vi "U3 AIN and PWM (ePut).vi"(9 "Timer0 Duty Cycle [%]":dbl=50.0 format="%.1f", 10 "16-bit PWM Frequency [Hz]":dbl=52.0 format="%.2f") -> (2 "Actual 16-bit Frequency":dbl format="%.1f")   [LabVIEW 2021]
panel:
  out "Timer0 Value":u16
  out "AIN0":dbl format="%_6g"
  in  "Timer/Counter Pin Offset":u8=4
  in  "stop":bool
  in  "FirstFound":bool=TRUE
  in  "Address":string="1"
  out "TimerClockDivisor":u8
  out "Error Message":string
  # "Demonstrates 1 channel of analog input with 1 channel of 16-bit PWM output.\nUses the 48 MHz divisor capable clock, and chooses a timer clock divisor to get\nas close as possible to the desired 16-bit PWM frequency.  Unlike \"U3 2-PWM.vi\",\nthis example updates the Timer0 Value every iteration even if it is the same.\nIf pin offset is 4, the PWM16 will be on FIO4."
  # "This example allows the duty cycle to\nbe changed while the VI is running."
  # "Range is 2.86 to 732.42 Hz"
  # "This VI passes a timer\nbase clock constant that\nis valid for hardware V1.21.\nFor hardware V1.20 change\nLJ_tc48MHZ_DIV to LJ_tc24MHZ_DIV."
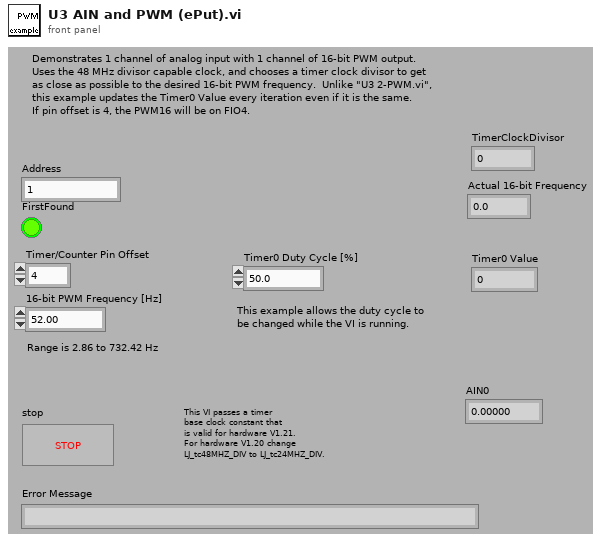
[diagram p1: front panel]
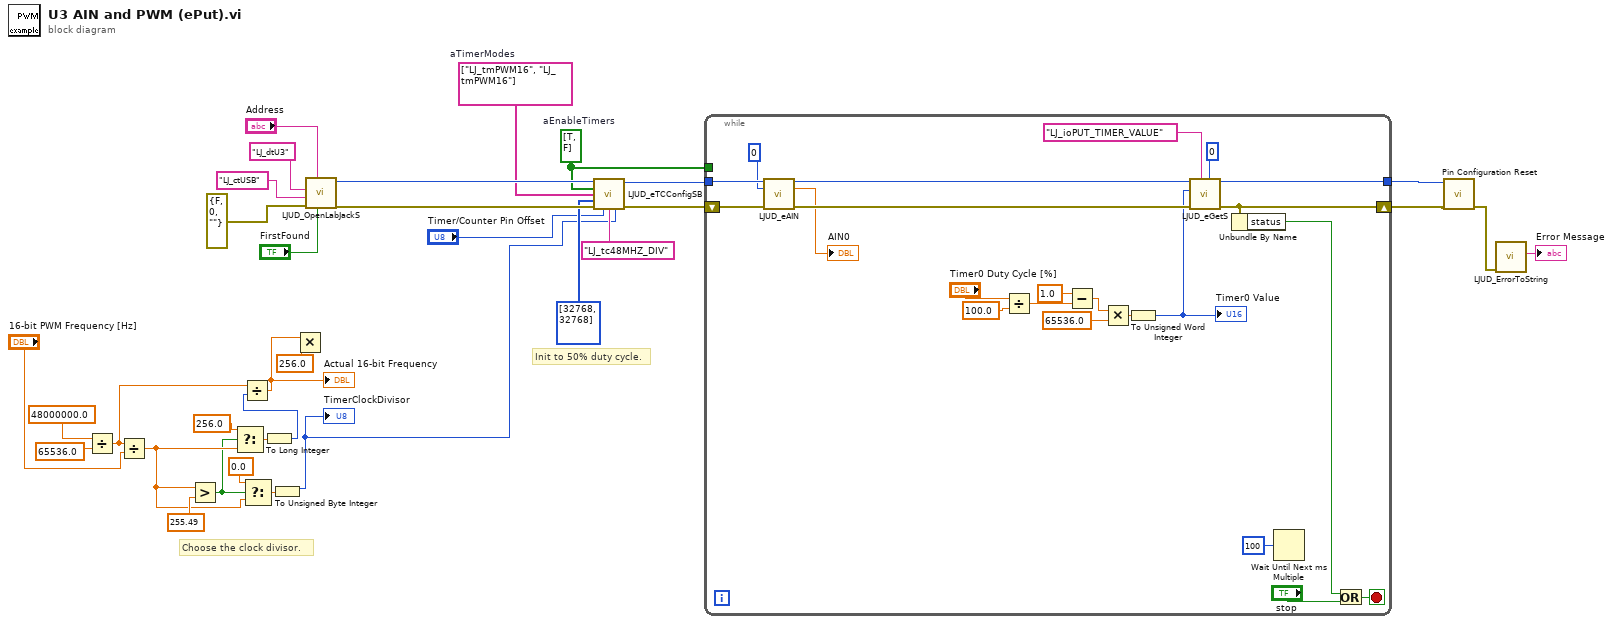
[diagram p0: block diagram]
diagram:
  w2 = bool[] [TRUE, FALSE]  # aEnableTimers
  w7 = string[] ["LJ_tmPWM16", "LJ_tmPWM16"]  # aTimerModes
  # "Choose the clock divisor."
  # "Init to 50% duty cycle."
  n1 = Divide(x=48000000.0, y=65536.0) -> (x/y=w21:dbl)
  n2 = Divide(x=w21, y="16-bit PWM Frequency [Hz]") -> (x/y=w25:dbl)
  n3 = Greater?(x=w25, y=255.49) -> (0:w24:bool)
  n4 = Select(t=256.0, s=w24, f=w25) -> (s? t:f=w27:dbl)
  n5 = Select(t=0.0, s=w24, f=w25) -> (s? t:f=w30:dbl)
  n6 = To Long Integer(number=w27) -> (32bit integer=w23:i32)
  n7 = Divide(x=w21, y=w23) -> (x/y=w20:dbl)
  "Actual 16-bit Frequency" <- w20
  n8 = To Unsigned Byte Integer(number=w30) -> (unsigned 8bit integer=w3:u8)
  "TimerClockDivisor" <- w3
  n9 = Multiply(x=w20, y=256.0) -> ()  [unwired: 1 out]
  n10 = call "LJUD_OpenLabJackS.vi"("FirstFound"="FirstFound", "Address"="Address", "error in"=errorcluster {"status"=FALSE, "code"=0, "source"=""}, "ConnectionType"="LJ_ctUSB", "DeviceType"="LJ_dtU3") -> ("error out"=w8:errorcluster, "Handle"=w9:i32)  [unwired: 4 in, 1 out]
  n11 = call "LJUD_eTCConfigSB.vi"("Handle In"=w9, "aEnableTimers"=w2, "aTimerModes"=w7, "aTimerValues"=u16[] [32768, 32768] ("TimerValues"), "error in"=w8, "TCPinOffset"="Timer/Counter Pin Offset", "TimerClockBase"="LJ_tc48MHZ_DIV" ("Timer Clock Base"), "TimerClockDivisor"=w3) -> ("Handle Out"=w10:i32, "error out"=w11:errorcluster)  [unwired: 6 in]
  n12 = while {
    tunnel: w2 -> [_]
    tunnel: [w44] -> w18
    tunnel: w10 -> [w42]
    shift-left: w11 -> [w41]
    shift-right: [w43] -> w17
    stop <- w48 stop-if-true
    n13 = call "LJUD_eAIN.vi"("Handle In"=w42, "ChannelP"=0, "error in"=w41) -> ("Handle Out"=w39:i32, "Voltage"=→"AIN0":dbl, "error out"=w40:errorcluster)  [unwired: 10 in]
    n14 = Divide(x="Timer0 Duty Cycle [%]", y=100.0) -> (x/y=w53:dbl)
    n15 = Subtract(x=1.0, y=w53) -> (x-y=w51:dbl)
    n16 = Multiply(x=w51, y=65536.0) -> (x*y=w50:dbl)
    n17 = To Unsigned Word Integer(number=w50) -> (unsigned 16bit integer=w36:u16)
    "Timer0 Value" <- w36
    n18 = call "LJUD_eGetS.vi"("Channel"=0, "IOType"="LJ_ioPUT_TIMER_VALUE", "error in"=w40, "Value Write"=w36, "Handle In"=w39) -> ("error out"=w43:errorcluster, "Handle Out"=w44:i32)  [unwired: 4 in, 1 out]
    n19 = Unbundle By Name(w43) -> ("status"=w47:bool)
    n20 = Wait Until Next ms Multiple(millisecond multiple=u32 100) -> ()  [unwired: 1 out]
    n21 = Or(x=w47, y="stop") -> (x .or. y?=w48:bool)
  }
  n22 = call "Pin Configuration Reset.vi"("error in"=w17, "Handle In"=w18) -> ("error out"=w16:errorcluster)  [unwired: 8 in, 1 out]
  n23 = call "LJUD_ErrorToString.vi"("error in"=w16) -> ("String"=→"Error Message":string)  [unwired: 10 in]
